vi "Shoot Speed Convert.vi"(2 "Shooter speed in (u/100ms)":dbl, 3 "Shooter speed in (RPM)":dbl) -> (0 "Shooter Speed out (RPM)":dbl, 1 "Shooter Speed out (u/100ms)":dbl)   [LabVIEW 2019]
panel:
  # "Will need to update if motor: shooter wheel ratio is not 1:1"
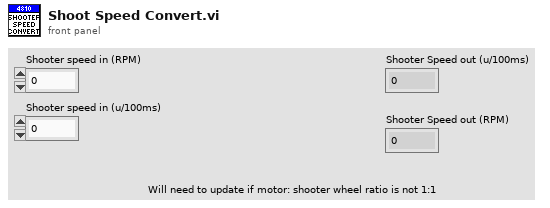
[diagram p1: front panel]
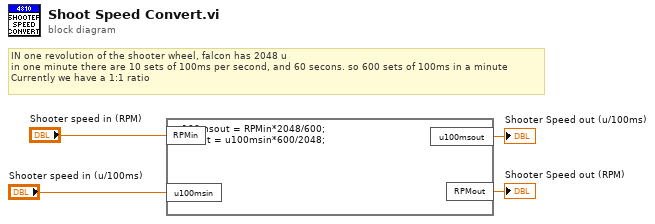
[diagram p0: block diagram]
diagram:
  # "IN one revolution of the shooter wheel, falcon has 2048 u \nin one minute there are 10 sets of 100ms per second, and 60 secons. so 600 sets of 100ms in a minute \nCurrently we have a 1:1 ratio"
  n1 = formula code="u100msout = RPMin*2048/600;\nRPMout = u100msin*600/2048;"("RPMin"="Shooter speed in (RPM)", "u100msin"="Shooter speed in (u/100ms)") -> ("u100msout"=→"Shooter Speed out (u/100ms)":dbl, "RPMout"=→"Shooter Speed out (RPM)":dbl)
